vi "OpenFont.vi"(8 "No Error":errorcluster, 10 "Pt Size":sgl, 11 "File":path) -> (0 "error out":errorcluster, 3 "Font [TTF_Font *]":i64 format="%.0x")   [LabVIEW 2024, in "SDL3.lvlib" / "TTF.lvlib"]
doc: "<B>Summary</B>\nCreate a font from a file, using a specified point size.\n\n<B>Remarks</B>\nSome .fon fonts will have several sizes embedded in the file, so the point size becomes the index of choosing which size. If the value is too high, the last indexed size will be the default.\n\nWhen done with the returned <B>TTF_Font</B>, use <B>TTF_CloseFont()</B> to dispose of it."
uses:
  TTF.lvlib
  <vilib>/Utility/error.llb/Error Cluster From Error Code.vi
  Lib/Win32/SDL3_ttf.dll
  Error/Error.lvlib
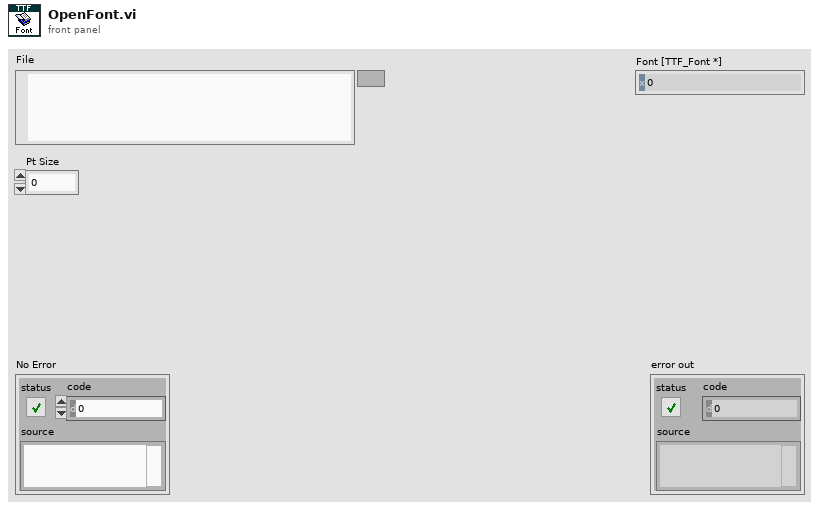
[diagram p1: front panel]
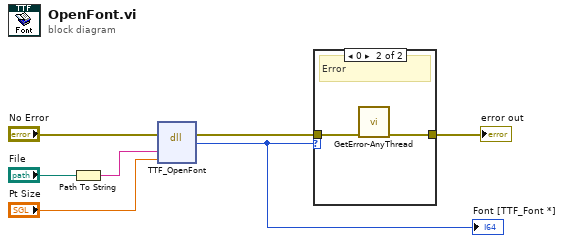
[diagram p0: block diagram]
diagram:
  n1 = Path To String(path="File") -> (string=w3:string)
  n2 = dll-call lib="C:/Users/Thomas/Documents/Projects/LV-SDL3/Lib/Win32/SDL3_ttf.dll" fn="TTF_OpenFont"(error in="No Error", "file"=w3, "ptsize"="Pt Size") -> (error out=w5:errorcluster, "return type"=w1:i64)  [unwired: 4 in, 1 out]
  "Font [TTF_Font *]" <- w1
  n3 = case shown="0" w1 {
    tunnel: w5 -> [w8 w10]
    tunnel: [w8 w9] -> w6
    frame Default {
      # "Ok"
    }
    frame 0 {
      # "Error"
      n4 = call "GetError-AnyThread.vi"("No Error"=w10) -> ("Error Out"=w9:errorcluster)  [unwired: 10 in]
    }
  }
  "error out" <- w6
